vi "tx_server.vi"() -> ()   [LabVIEW 2020]
uses:
  <vilib>/addons/Modulation/Digital/General/MT Generate PSK System Parameters(M).vi
  <instrlib>/niUSRP/niUSRP Write Tx Data (CDB Cluster).vi
  <vilib>/addons/Modulation/niDMT.lvlib
panel:
  in  "Tab Control":T1(tab)
  out "return value":string
  in  "module path":path
  in  "Packet Parameters":T2={"Guard Bits "=30, "Sync Bits"=20, "Message Bits"=128}
  in  "Packet Pad \n[samples]":i32=200
  in  "Blank Frame \n[samples]":i32=500
  out "Number of Packets in Message":i32=46
  in  "PN sequence order\nfor Sync Bits":i32=31 caption="PN sequence order (9)"
  in  "Packet Repeat":i32=2
  in  "Select PSK Modulation Format":T3(tab)=enum."QPSK" caption="PSK"
  in  "BPSK System Parameters":T4={"Samples per Symbol"=8, "symbol map"=[], "Differential PSK"=enum."disable", "PSK type"=0} {"PSK type" items=["normal", "shifted", "offset"]; "symbol map" format="%.3f"}
  in  "QPSK System Parameters":T4={"Samples per Symbol"=8, "symbol map"=[], "Differential PSK"=enum."disable", "PSK type"=0} {"PSK type" items=["normal", "shifted", "offset"]; "symbol map" format="%.3f"}
  in  "pi/4 DQPSK System Parameters":T4={"Samples per Symbol"=8, "symbol map"=[], "Differential PSK"=enum."enable", "PSK type"=1} {"PSK type" items=["normal", "shifted", "offset"]; "symbol map" format="%.3f"}
  in  "OQPSK System Parameters":T4={"Samples per Symbol"=8, "symbol map"=[], "Differential PSK"=enum."disable", "PSK type"=2} {"PSK type" items=["normal", "shifted", "offset"]; "symbol map" format="%.3f"}
  in  "8-PSK System Parameters":T4={"Samples per Symbol"=8, "symbol map"=[], "Differential PSK"=enum."disable", "PSK type"=0} {"PSK type" items=["normal", "shifted", "offset"]; "symbol map" format="%.3f"}
  in  "16-PSK System Parameters":T4={"Samples per Symbol"=8, "symbol map"=[], "Differential PSK"=enum."disable", "PSK type"=0} {"PSK type" items=["normal", "shifted", "offset"]; "symbol map" format="%.3f"}
  in  "M":i32=4 min=2 step=2
  in  "Custom System Parameters":T4={"Samples per Symbol"=8, "symbol map"=[], "Differential PSK"=enum."disable", "PSK type"=0} {"PSK type" items=["normal", "shifted", "offset"]; "symbol map" format="%.3f"}
  in  "Pulse Shaping Filter Parameters":T5={"Alpha"=0.5, "Filter Length"=6, "TX Filter"=enum."Root Raised Cos"} caption="Pulse Shaping Filter" {"Alpha" format="%.2f"}
  in  "Tx Parameters":T6={"Tx IQ Sampling\nRate [s/sec]"=500000.0, "Tx Frequency [Hz]"=2500000000.0, "Tx Gain [dB]"=0.0, "Tx Antenna"="TX1"} {"Tx Gain [dB]" format="%#.6p"; "Tx Frequency [Hz]" format="%#.6p"; "Tx IQ Sampling\nRate [s/sec]" format="%#.6p"}
  out "Actual Tx Parameters":T6={"Tx IQ Sampling\nRate [s/sec]"=200000.0, "Tx Frequency [Hz]"=2500000000.0, "Tx Gain [dB]"=0.0, "Tx Antenna"="TX1"} {"Tx Gain [dB]" format="%#.6p"; "Tx Frequency [Hz]" format="%#.6p"; "Tx IQ Sampling\nRate [s/sec]" format="%#.6p"}
  in  "USRP IP address":refnum<k15>="192.168.10.2"
  out "error out":errorcluster
  in  "Queue Length":i32=10
  out "Constellation Graph":T7(graph)
  in  "autoscale":bool
  out "Symbol Rate\n[symbols/sec]":dbl=25000.0 format="%#.6p"
  in  "stop":bool
  # "Guard\nBand"
  # "Sync\nSeq"
  # "Packet\nNumber"
  # "Pad\nData"
  # "Blank\nFrame"
  # "Data"
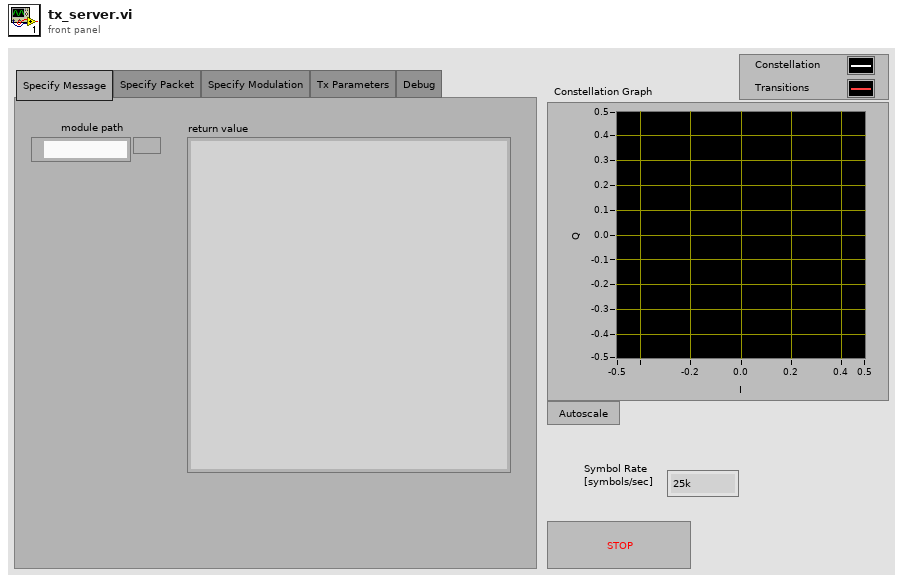
[diagram p1: front panel]
types:
  T1 = enum32{"Specify Message", "Specify Packet", "Specify Modulation", "Tx Parameters", "Debug"}
  T2 = cluster{"Guard Bits ":i32, "Sync Bits":i32, "Message Bits":i32}
  T3 = enum32{"BPSK", "QPSK", "pi/4DQPSK", "OQPSK", "8-PSK", "16-PSK", "Custom"}
  T4 = cluster{"Samples per Symbol":i32, "symbol map":cdb[], "Differential PSK":enum16{"disable", "enable"}, "PSK type":u16}
  T5 = cluster{"Alpha":dbl, "Filter Length":i32, "TX Filter":enum16{"none", "Raised Cosine", "Root Raised Cos", "Gaussian"}}
  T6 = cluster{"Tx IQ Sampling\nRate [s/sec]":dbl, "Tx Frequency [Hz]":dbl, "Tx Gain [dB]":dbl, "Tx Antenna":string}
  T7 = cluster{"Decimated Array":dbl[], "Decimated Array":dbl[]}[]
  T8 = cluster{"samples per symbol (16)":i32, "symbol map":cdb[], "differential PSK":enum16{"disable", "enable"}, "PSK type":u16}
  T9 = cluster{"s? t:f":cluster{"t0":dbl, "dt":dbl, "Y":cdb[]}, i32}
  T10 = cluster{"output complex waveform":cluster{"t0":dbl, "dt":dbl, "Y":cdb[]}, i32}
  T11 = cluster{"constellation":dbl[], "oversampled data":dbl[]}[]
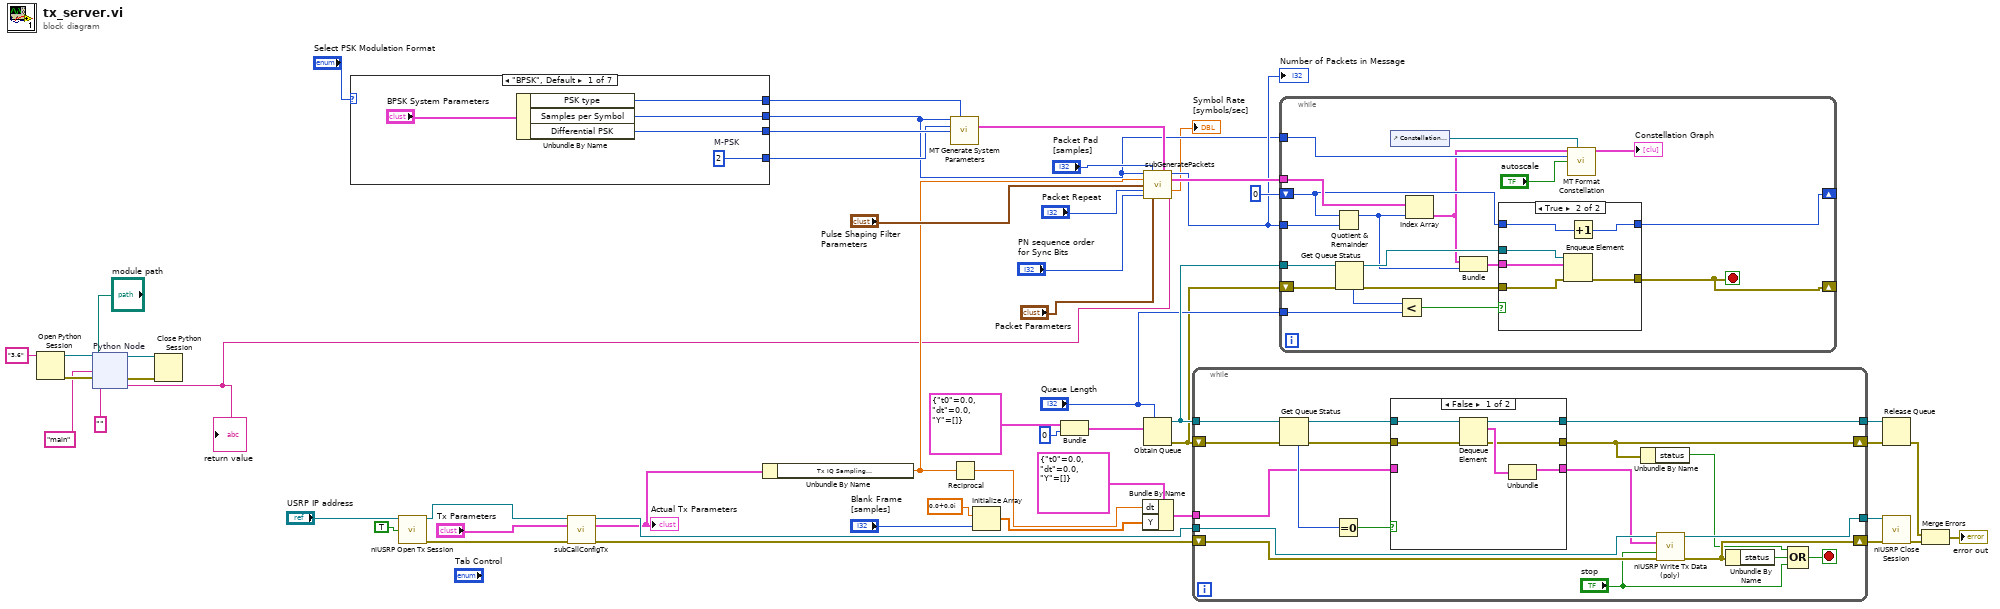
[diagram p0: block diagram]
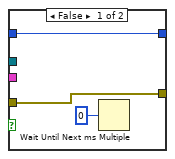
[diagram p2: hidden frame]
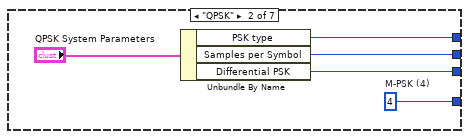
[diagram p3: hidden frame]
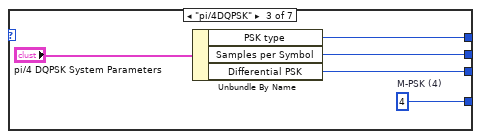
[diagram p4: hidden frame]
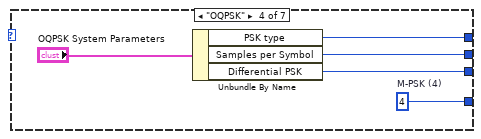
[diagram p5: hidden frame]
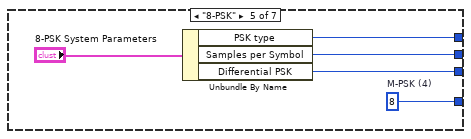
[diagram p6: hidden frame]
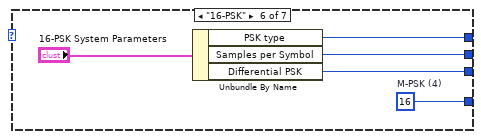
[diagram p7: hidden frame]
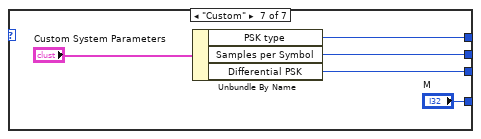
[diagram p8: hidden frame]
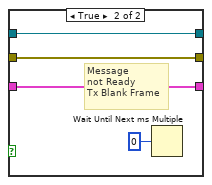
[diagram p9: hidden frame]
diagram:
  n1 = Open Python Session(python version="3.6" ("Python version")) -> (session out=w8:refnum<k35>, error out=w6:errorcluster)  [unwired: 2 in]
  n2 = node "Python Node"(w8, "module path", "main" ("function name"), w6, "") -> (w7:refnum<k35>, w5:errorcluster, w2:string)  [unwired: 2 out]
  "return value" <- w2
  n3 = Close Python Session(session in=w7, error in=w5) -> ()  [unwired: 1 out]
  n4 = case shown="\"BPSK\", Default" "Select PSK Modulation Format" {
    tunnel: [w54 w58 w66 w71 w76 w82 w85] -> w12
    tunnel: [w55 w60 w65 w70 w75 w81 w86] -> w51
    tunnel: [w57 w62 w67 w72 w74 w80 "M"] -> w33
    tunnel: [w56 w61 w64 w69 w77 w79 w87] -> w20
    frame "BPSK", Default {
      w57 = 2  # M-PSK
      n5 = Unbundle By Name("BPSK System Parameters") -> ("PSK type"=w56:u16, "Samples per Symbol"=w54:i32, "Differential PSK"=w55:enum16{"disable", "enable"})
    }
    frame "QPSK" {
      w62 = 4  # M-PSK (4)
      n6 = Unbundle By Name("QPSK System Parameters") -> ("PSK type"=w61:u16, "Samples per Symbol"=w58:i32, "Differential PSK"=w60:enum16{"disable", "enable"})
    }
    frame "pi/4DQPSK" {
      w67 = 4  # M-PSK (4)
      n7 = Unbundle By Name("pi/4 DQPSK System Parameters") -> ("PSK type"=w64:u16, "Samples per Symbol"=w66:i32, "Differential PSK"=w65:enum16{"disable", "enable"})
    }
    frame "OQPSK" {
      w72 = 4  # M-PSK (4)
      n8 = Unbundle By Name("OQPSK System Parameters") -> ("PSK type"=w69:u16, "Samples per Symbol"=w71:i32, "Differential PSK"=w70:enum16{"disable", "enable"})
    }
    frame "8-PSK" {
      w74 = 8  # M-PSK (4)
      n9 = Unbundle By Name("8-PSK System Parameters") -> ("PSK type"=w77:u16, "Samples per Symbol"=w76:i32, "Differential PSK"=w75:enum16{"disable", "enable"})
    }
    frame "16-PSK" {
      w80 = 16  # M-PSK (4)
      n10 = Unbundle By Name("16-PSK System Parameters") -> ("PSK type"=w79:u16, "Samples per Symbol"=w82:i32, "Differential PSK"=w81:enum16{"disable", "enable"})
    }
    frame "Custom" {
      n11 = Unbundle By Name("Custom System Parameters") -> ("PSK type"=w87:u16, "Samples per Symbol"=w85:i32, "Differential PSK"=w86:enum16{"disable", "enable"})
    }
  }
  n12 = call <instrlib>:"niUSRP Open Tx Session.vi"("device names"="USRP IP address", "reset"=TRUE) -> ("session handle out"=w24:refnum<k15>, "error out"=w23:errorcluster)  [unwired: 12 in]
  n13 = call "subCallConfigTx.vi"("session handle"=w24, "Tx Parameters"="Tx Parameters", "error in"=w23) -> ("session handle out"=w32:refnum<k15>, "Actual Tx Parameters"=w31:T6, "error out"=w37:errorcluster)  [unwired: 10 in]
  "Actual Tx Parameters" <- w31
  n14 = Unbundle By Name(w31) -> ("Tx IQ Sampling\nRate [s/sec]"=w13:dbl)
  n15 = call-poly <vilib>:"MT Generate System Parameters.vi"("samples per symbol (16)"=w12, "PSK type"=w20, "M-PSK (4)"=w33, "differential PSK"=w51) -> ("PSK system parameters"=w21:T8)  [unwired: 9 in, 2 out]
  n16 = Reciprocal(x=w13) -> (1/x=w34:dbl)
  n17 = Initialize Array(cdb 0.0+0.0i ("element"), "Blank Frame \n[samples]") -> (w47:cdb[])
  n18 = Bundle("s? t:f"=cluster{"t0":dbl, "dt":dbl, "Y":cdb[]} {"t0"=0.0, "dt"=0.0, "Y"=[]}, 0) -> (w42:T9)  [unwired: 1 in]
  n19 = Bundle By Name(cluster=cluster{"t0":dbl, "dt":dbl, "Y":cdb[]} {"t0"=0.0, "dt"=0.0, "Y"=[]} ("s? t:f"), "dt"=w34, "Y"=w47) -> (w46:cluster{"t0":dbl, "dt":dbl, "Y":cdb[]})
  n20 = call "subGeneratePackets.vi"("Samples per Symbol"=w12, "Packet Pad \n[samples]"="Packet Pad \n[samples]", "PSK system parameters"=w21, "Tx IQ Sampling\nRate [s/sec]"=w13, "Pulse Shaping Filter Parameters"="Pulse Shaping Filter Parameters", "Packet Repeat"="Packet Repeat", "PN sequence order\nfor Sync Bits"="PN sequence order\nfor Sync Bits", "Packet Parameters"="Packet Parameters", "Message Text"=w2) -> ("Number of Packets"=w30:i32, "Packets"=w39:cluster{"t0":dbl, "dt":dbl, "Y":cdb[]}[], "Symbol Rate"=→"Symbol Rate\n[symbols/sec]":dbl)  [unwired: 4 in]
  "Number of Packets in Message" <- w30
  n21 = Obtain Queue(max queue size (-1, unlimited)="Queue Length", element data type=w42) -> (queue out=w48:refnum<queue>, error out=w26:errorcluster)  [unwired: 3 in, 1 out]
  n22 = while {
    tunnel: w32 -> [w96]
    shift-right: [w93] -> w36
    shift-left: w37 -> [w97]
    tunnel: w48 -> [w105]
    tunnel: w46 -> [w102]
    tunnel: [w101] -> w45
    tunnel: [w95] -> w35
    shift-right: [w90] -> w44
    shift-left: w26 -> [w98]
    stop <- w92 stop-if-true
    n23 = Get Queue Status(queue=w105, error in (no error)=w98) -> (queue out=w100:refnum<queue>, error out=w99:errorcluster, # elements in queue=w104:i32)  [unwired: 1 in, 5 out]
    n24 = Equal To 0?(x=w104) -> (x = 0?=w103:bool)
    n25 = case shown="False" w103 {
      tunnel: w102 -> [_ w115]
      tunnel: [w107 w115] -> w88
      tunnel: [w111 w113] -> w101
      tunnel: [w106 w114] -> w90
      tunnel: w100 -> [w110 w113]
      tunnel: w99 -> [w109 w114]
      frame False {
        n26 = Dequeue Element(queue=w110, error in (no error)=w109) -> (queue out=w111:refnum<queue>, element=w108:T9, error out=w106:errorcluster)  [unwired: 1 in, 1 out]
        n27 = Unbundle(w108) -> ("s? t:f"=w107:cluster{"t0":dbl, "dt":dbl, "Y":cdb[]})  [unwired: 1 out]
      }
      frame True {
        # "Message\nnot Ready\nTx Blank Frame"
        n28 = Wait Until Next ms Multiple(millisecond multiple=u32 0) -> ()  [unwired: 1 out]
      }
    }
    n29 = Unbundle By Name(w90) -> ("status"=w89:bool)
    n30 = call-poly <instrlib>:"niUSRP Write Tx Data (poly).vi"("session handle"=w96, "data"=w88, "end of data?"="stop", "error in (no error)"=w97) -> ("session handle out"=w95:refnum<k15>, "error out"=w93:errorcluster)  [unwired: 10 in]
    n31 = Unbundle By Name(w93) -> ("status"=w94:bool)
    n32 = Compound Arithmetic op=OR(w89, w94, "stop") -> (w92:bool)
  }
  n33 = while {
    tunnel: w48 -> [w134]
    shift-right: [w127] -> _
    shift-left: 0 -> [w123]
    tunnel: w39 -> [w124]
    tunnel: "Queue Length" -> [w126]
    tunnel: w30 -> [w125]
    shift-right: [w121] -> _
    shift-left: w26 -> [w129]
    tunnel: w12 -> [w118]
    stop <- w121 stop-if-true
    n34 = Quotient & Remainder(x=w123, y=w125) -> (x-y*floor(x/y)=w122:i32)  [unwired: 1 out]
    n35 = Get Queue Status(queue=w134, error in (no error)=w129) -> (queue out=w133:refnum<queue>, error out=w130:errorcluster, # elements in queue=w132:i32)  [unwired: 1 in, 5 out]
    n36 = control-ref of="Constellation Graph"() -> (w119:refnum<vi>)
    n37 = Less?(x=w132, y=w126) -> (x < y?=w131:bool)
    n38 = Index Array(array=w124, index=w122) -> (element=w116:cluster{"t0":dbl, "dt":dbl, "Y":cdb[]})
    n39 = Bundle("output complex waveform"=w116, w122) -> (w128:T10)  [unwired: 1 in]
    n40 = case shown="True" w131 {
      tunnel: w130 -> [w135 w143]
      tunnel: w133 -> [_ w142]
      tunnel: [w135 w141] -> w121
      tunnel: w128 -> [_ w140]
      tunnel: w123 -> [w137 w139]
      tunnel: [w137 w138] -> w127
      frame False {
        n41 = Wait Until Next ms Multiple(millisecond multiple=u32 0) -> ()  [unwired: 1 out]
      }
      frame True {
        n42 = Enqueue Element(queue=w142, element=w140, error in (no error)=w143) -> (error out=w141:errorcluster)  [unwired: 1 in, 2 out]
        n43 = Increment(x=w139) -> (x+1=w138:i32)
      }
    }
    n44 = call <vilib>:"MT Format Constellation.vi"("waveform"=w116, "constellation reference"=w119, "samples per symbol"=w118, "autoscale"="autoscale") -> ("constellation graph"=→"Constellation Graph":T11)  [unwired: 1 in, 10 out]
  }
  n45 = Release Queue(queue=w45, error in (no error)=w44) -> (error out=w19:errorcluster)  [unwired: 3 out]
  n46 = call <instrlib>:"niUSRP Close Session.vi"("session handle"=w35, "error in (no error)"=w36) -> ("error out"=w18:errorcluster)  [unwired: 13 in]
  n47 = Merge Errors(w19, w18) -> (→"error out":errorcluster)
